vi "combineTxt.vi"(8 "error in (no error)":errorcluster caption="错误输入（无错误）", 10 "parentPath":path, 11 "childPath":path) -> (0 "error out":errorcluster)   [LabVIEW 2011]
uses:
  <vilib>/Utility/file.llb/Read From Spreadsheet File (string).vi
  <vilib>/Utility/file.llb/Write To Spreadsheet File (string).vi
  <vilib>/Utility/config.llb/NI_LVConfig.lvlib
panel:
  in  "xml_info":T1={"FileVersion"="DevelopmentSystem", "FileName"="DevelopmentSystem", "test time"=["2016/11/14 11:59:03"], "original Path"=path "D:/高频房软件/2. HPTS_VNA_Rev2.7.1.3-1107最新源码/Demo_data", "show_TDD11"=[], "show_TDD22"=[], "show_impspec"=[], "usedSN"="", "diffspec"={"limit Spec"=[], "Diff Test Item Name"=[], "Spec _Col"=[]}, "secondresult"=[], "show_Terminal Point"=[], "show_Cable Point"=[], "customerPN"="", "auto get refer point"=FALSE, "width1"=0, "width2"=0}
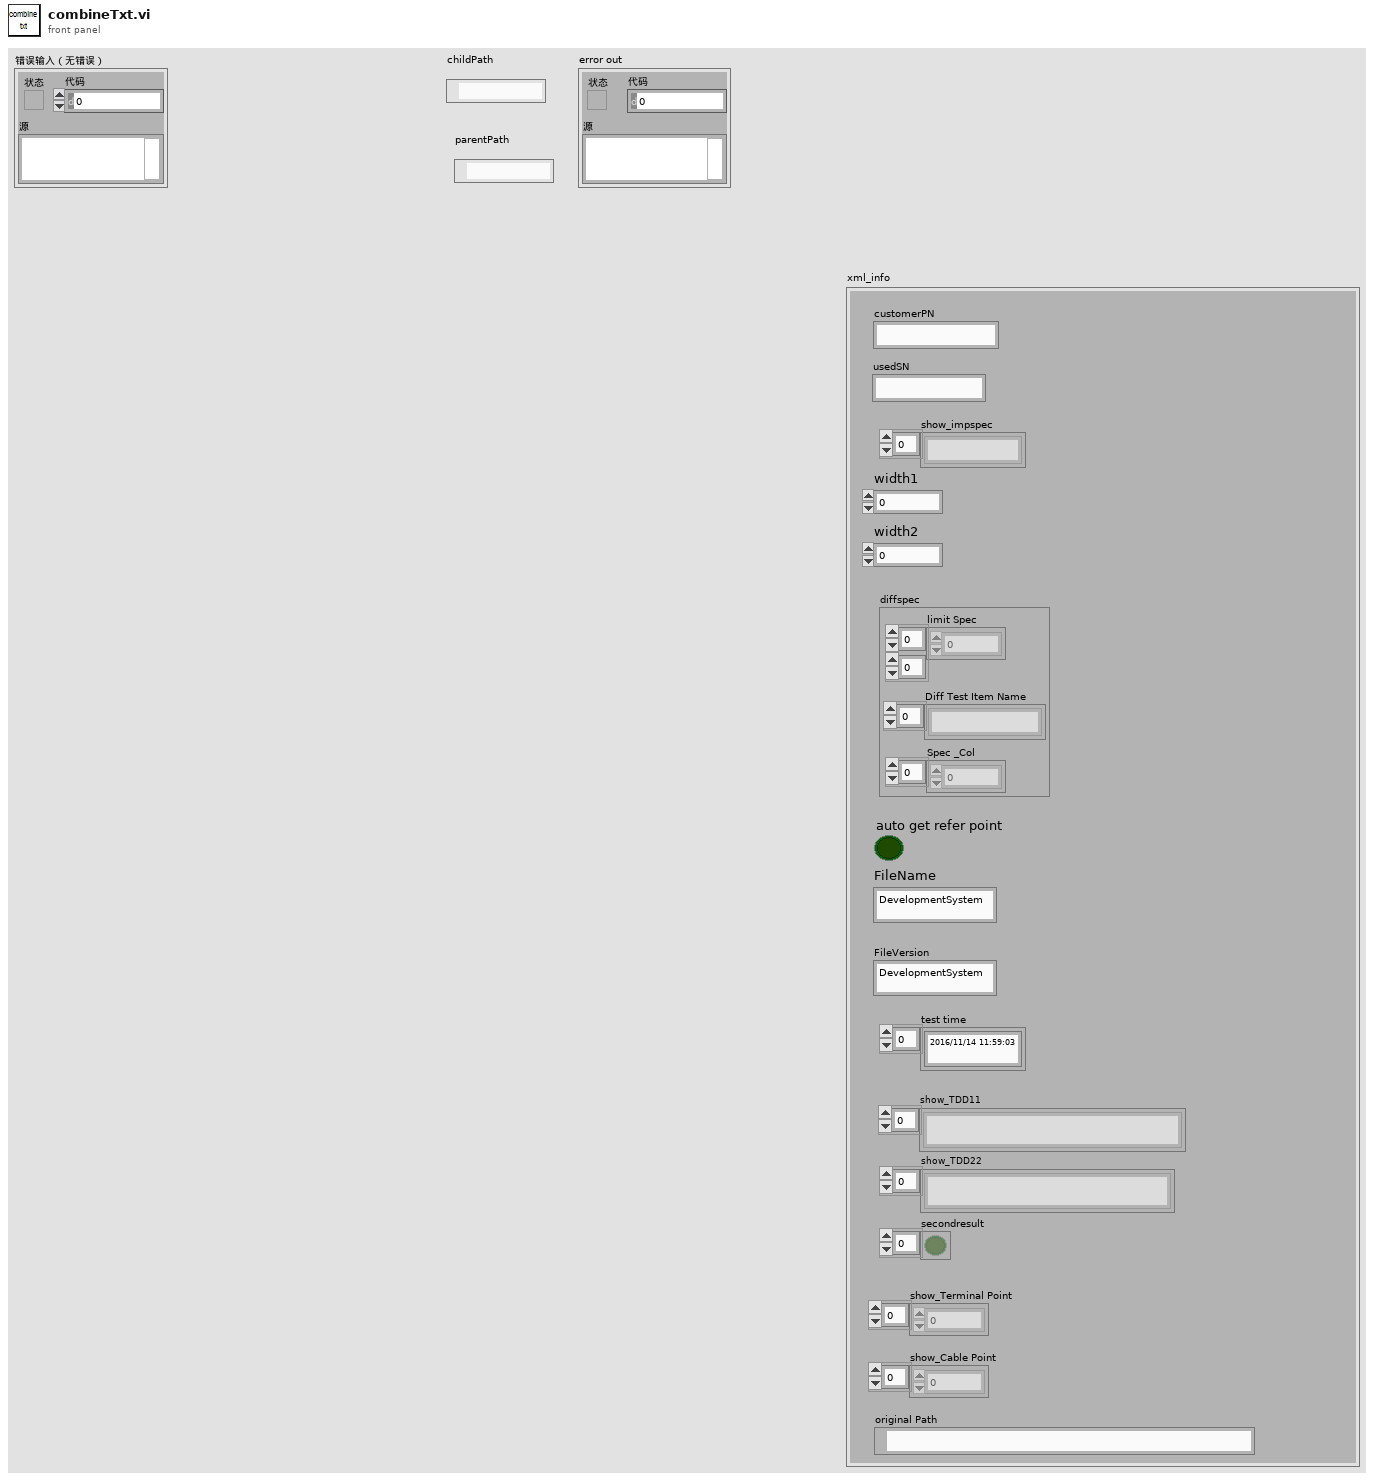
[diagram p1: front panel]
types:
  T1 = cluster{"FileVersion":string, "FileName":string, "test time":string[], "original Path":path, "show_TDD11":string[], "show_TDD22":string[], "show_impspec":string[], "usedSN":string, "diffspec":cluster{"limit Spec":dbl[][], "Diff Test Item Name":string[], "Spec _Col":i32[]}, "secondresult":bool[], "show_Terminal Point":dbl[], "show_Cable Point":dbl[], "customerPN":string, "auto get refer point":bool, "width1":i32, "width2":i32}
  T2 = typedef "NI_LVConfig.lvlib/Config Data RefNum.ctl" = refnum<k1>
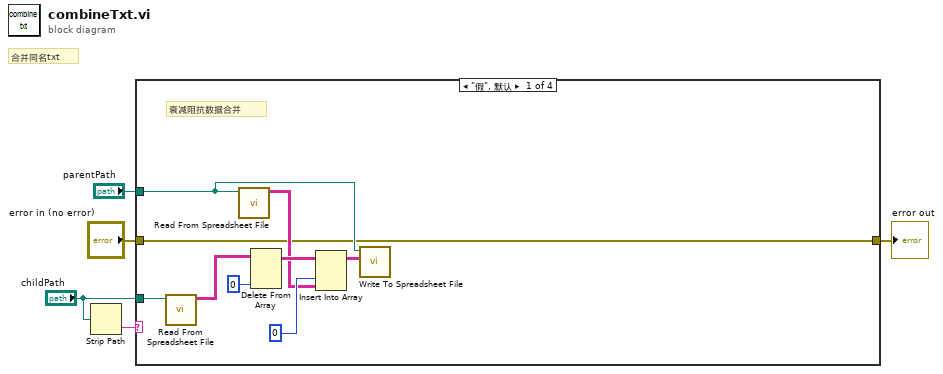
[diagram p0: block diagram]
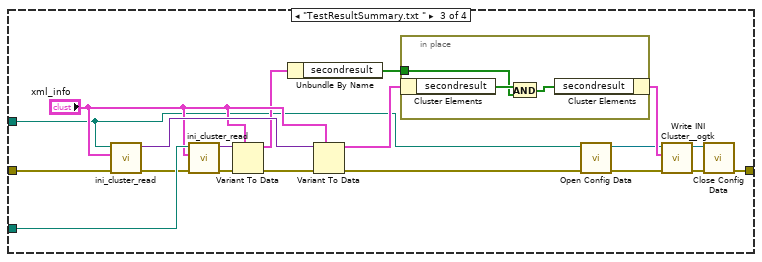
[diagram p3: hidden frame]
diagram:
  # "合并同名txt"
  n1 = Strip Path(path="childPath") -> (name=w5:string)  [unwired: 1 out]
  n2 = case shown="\"假\", 默认" w5 {
    tunnel: "childPath" -> [w14 _ w33 _]
    tunnel: "parentPath" -> [w7 _ w26 _]
    tunnel: "error in (no error)" -> [w6 w15 w20 w38]
    tunnel: [w6 w15 w16 w38] -> w1
    frame "假", Default {
      # "衰减阻抗数据合并"
      n3 = call-poly <vilib>:"Read From Spreadsheet File.vi"("file path (dialog if empty)"=w14) -> ("all rows"=w13:string[][])  [unwired: 6 in, 4 out]
      n4 = call-poly <vilib>:"Read From Spreadsheet File.vi"("file path (dialog if empty)"=w7) -> ("all rows"=w9:string[][])  [unwired: 6 in, 4 out]
      n5 = Delete From Array(array=w13, index (col)=0 ("禁用的索引 (列)")) -> (array with subset deleted=w11:string[][])  [unwired: 2 in, 1 out]
      n6 = Insert Into Array(array=w11, index (col)=0 ("禁用的索引 (列)"), new element=w9) -> (w8:string[][])  [unwired: 1 in]
      n7 = call-poly <vilib>:"Write To Spreadsheet File.vi"("2D data"=w8, "file path (dialog if empty)"=w7) -> ()  [unwired: 6 in, 1 out]
    }
    frame "EEPROMPort0.txt", "EEPROMPort1.txt", "EEPROMPort2.txt", "EEPROMPort3.txt", "EEPROMPort4.txt", "EEPROMPort5.txt" {
    }
    frame "TestResultSummary.txt " {
      n8 = call "ini_cluster_read.vi"("error in (no error)"=w20, "INI Fomatted Cluster Type"="xml_info", "configuration file path"=w26) -> ("error out"=w23:errorcluster, "ini cluster out"=w32:variant)  [unwired: 7 in]
      n9 = call "ini_cluster_read.vi"("error in (no error)"=w23, "INI Fomatted Cluster Type"="xml_info", "configuration file path"=w33) -> ("error out"=w22:errorcluster, "ini cluster out"=w34:variant)  [unwired: 7 in]
      n10 = Variant To Data(error in=w22, type="xml_info", Variant=w34) -> (data=w30:T1, error out=w21:errorcluster)
      n11 = Unbundle By Name(w30) -> ("secondresult"=w28:bool[])
      n12 = Variant To Data(error in=w21, type="xml_info", Variant=w32) -> (data=w29:T1, error out=w19:errorcluster)
      n13 = in-place {
        in-place-border: w28 -> [w36]
        n14 = in-place-cluster #1(w29) -> ("secondresult"=w37:bool[])
        n15 = And(x=w37, y=w36) -> (x .and. y?=w35:bool[])
        n16 = in-place-cluster #1("secondresult"=w35) -> (w27:T1)
      }
      n17 = call <vilib>:"Open Config Data.vi"("error in (no error)"=w19, "configuration file path"=w26) -> ("error out"=w18:errorcluster, "refnum"=w25:T2)  [unwired: 7 in, 1 out]
      n18 = call <userlib>:"Write INI Cluster__ogtk.vi"("error in (no error)"=w18, "INI Fomatted Cluster"=w27, "refnum"=w25) -> ("error out"=w17:errorcluster, "dup refnum"=w24:T2)  [unwired: 7 in]
      n19 = call <vilib>:"Close Config Data.vi"("error in (no error)"=w17, "refnum"=w24) -> ("error out"=w16:errorcluster)  [unwired: 8 in, 1 out]
    }
    frame "xml_info.txt" {
    }
  }
  "error out" <- w1
